vi "Boiler Controller.vi"(8 "error in (no error)":errorcluster, 11 "Message Queues":T1) -> (0 "error out":errorcluster)   [LabVIEW 2015]
uses:
  support/Message Queue/All Message Queues.ctl
  support/Message Queue/Message Cluster.ctl
  support/Message Queue/Message Queue.lvlib
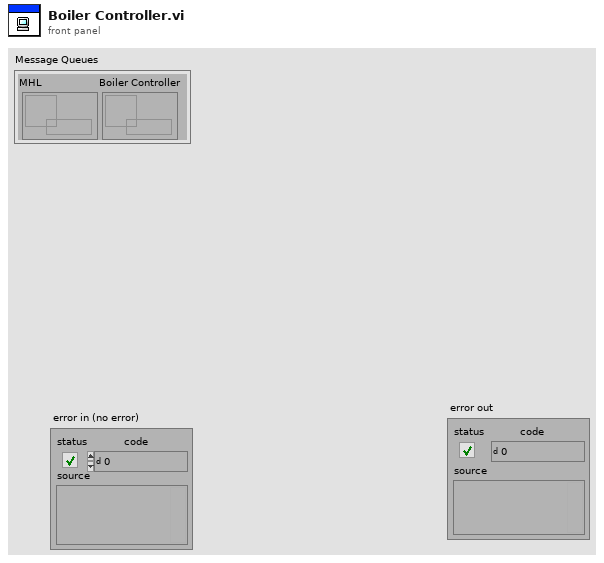
[diagram p1: front panel]
types:
  T1 = typedef "Message Queue.lvlib/All Message Queues.ctl" = cluster{"MHL":refnum<queue>, "Boiler Controller":refnum<queue>}
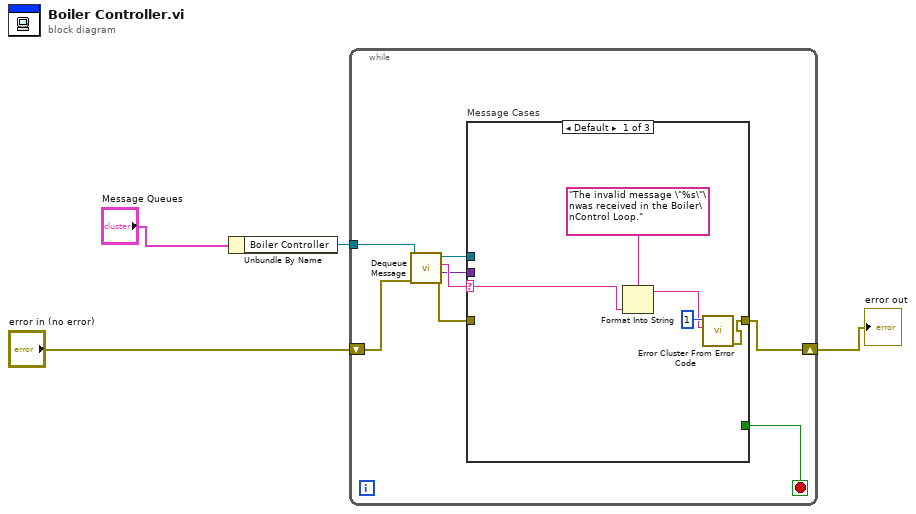
[diagram p0: block diagram]
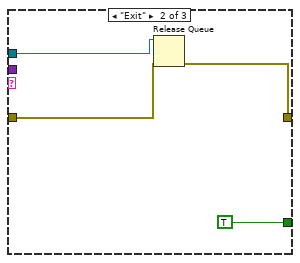
[diagram p2: hidden frame]
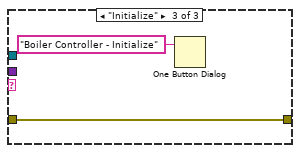
[diagram p3: hidden frame]
diagram:
  n1 = Unbundle By Name("Message Queues") -> ("Boiler Controller"=w2:refnum<queue>)
  n2 = while {
    tunnel: w2 -> [w12]
    shift-right: [w7] -> w1
    shift-left: "error in (no error)" -> [w11]
    stop <- w5 stop-if-true
    n3 = call "Dequeue Message.vi"("error in (no error)"=w11, "Message Queue"=w12) -> ("error out"=w8:errorcluster, "Message Data"=w9:variant, "Message"=w10:string, "dup Message Queue"=w6:refnum<queue>)  [unwired: 6 in]
    n4 = case "Message Cases" shown="Default" w10 {
      selector: w10 -> [w17 _ _]
      tunnel: w9 -> [_ _ _]
      tunnel: w8 -> [_ w20 w23]
      tunnel: [w15 w19 w23] -> w7
      tunnel: w6 -> [_ w21 _]
      tunnel: [_ TRUE _] -> w5
      frame Default {
        n5 = Format Into String(format string="The invalid message \"%s\"\nwas received in the Boiler\nControl Loop.", w17) -> (resulting string=w13:string)  [unwired: 2 in, 1 out]
        n6 = call <vilib>:"Error Cluster From Error Code.vi"("error message (\"\")"=w13, "error code (0)"=1) -> ("error out"=w15:errorcluster)  [unwired: 7 in]
      }
      frame "Exit" {
        n7 = Release Queue(queue=w21, error in (no error)=w20) -> (error out=w19:errorcluster)  [unwired: 1 in, 2 out]
      }
      frame "Initialize" {
        n8 = One Button Dialog(message="Boiler Controller - Initialize") -> ()  [unwired: 1 in, 1 out]
      }
    }
  }
  "error out" <- w1
